vi "Frequency_Plot_Builder.vi"() -> ()   [LabVIEW 2011]
panel:
  in  "Plot Data Destination":path
  in  "Data Folder":path
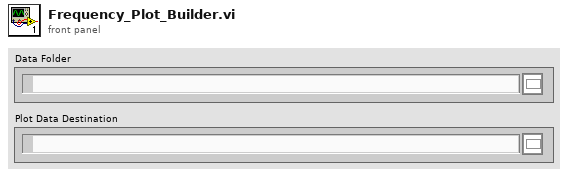
[diagram p1: front panel]
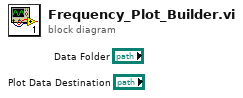
[diagram p0: block diagram]
diagram:
